vi "main(Test DQMH modules).bak.vi"() -> ()   [LabVIEW 2018, in "Application.lvlib"] (continued)
      frame "Test DRV 55" {
        w5444 = 55  # DUT index(0-59)
        n2417 = disable-structure shown="LOGGING==TRUE" {
          disable-tunnel: w5445 -> [w5480 _]
          frame condition #0 (active) {
            n2418 = Empty String/Path?(string/path=w5480) -> (empty?=w5483:bool)
            n2419 = Select(t="Quece timeout", s=w5483, f=w5480) -> (s? t:f=w5479:string)
            n2420 = call "string log (SubVI).vi"("Enum"=enum16{"Init", "Log", "Read"}."Log", "state Name"=w5479) -> ()  [unwired: 8 in, 2 out]
          }
          frame condition #1 {
          }
        }
        n2421 = call "progress string(SubVI).vi"("String 3"=w5445, "String in"=w5446) -> ("String out"=w5447:string)  [unwired: 9 in]
        n2422 = call "FGV Driver Data.vi"("DUT index(1-60)"=w5444) -> ("DUT SC"=w5443:bool)  [unwired: 7 in, 3 out]
        n2423 = case shown="False" w5443 {
          tunnel: [w5472 _] -> w5452
          tunnel: w5449 -> [w5471 _]
          frame False {
            w5459 = T11 {"command"="", "command data"=variant} ("element")
            w5458 = "MEAS.mux6_1"
            n2424 = To Variant(anything=T4."mux6-1_channel0" ("mux6_1(3wires)_encode")) -> (Variant=w5457:variant)
            n2425 = To Variant(anything=T4."mux6_1_channel1_3" ("mux6_1(3wires)_encode")) -> (Variant=w5469:variant)
            n2426 = To Variant(anything=T4."mux6-1_channel1_2" ("mux6_1(3wires)_encode")) -> (Variant=w5467:variant)
            n2427 = Bundle By Name(cluster=w5459, "command"=w5458, "command data"=w5467) -> (w5466:T11)
            n2428 = Bundle By Name(cluster=w5459, "command"=w5458, "command data"=w5469) -> (w5465:T11)
            n2429 = Bundle By Name(cluster=w5459, "command"=w5458, "command data"=w5457) -> ()  [unwired: 1 out]
            n2430 = Bundle By Name(cluster=w5459, "command"="MEAS.DMM dual read") -> (w5463:T11)
            n2431 = Build Array(w5466, w5465, w5463) -> (w5461:T11[])
            n2432 = Reverse 1D Array(array=w5461) -> (reversed array=w5462:T11[])
            n2433 = for {
              tunnel: [w5478] -> w5472 mode=indexing
              tunnel: w5471 -> [w5477]
              tunnel: w5462 -> [w5476] mode=indexing
              n2434 = Unbundle By Name(w5476) -> ("command"=w5475:string, "command data"=w5474:variant)
              n2435 = call "App enquece.vi"("Priority Enquece"=TRUE, "command data"=w5474, "command"=w5475, "queue in"=w5477) -> ("error out"=w5478:errorcluster)  [unwired: 6 in, 1 out]
            }
          }
          frame True {
          }
        }
        n2436 = Merge Errors(w5450, w5452) -> (w5451:errorcluster)
      }
      frame "Test DRV 56" {
        w5485 = 56  # DUT index(0-59)
        n2437 = disable-structure shown="LOGGING==TRUE" {
          disable-tunnel: w5486 -> [w5521 _]
          frame condition #0 (active) {
            n2438 = Empty String/Path?(string/path=w5521) -> (empty?=w5524:bool)
            n2439 = Select(t="Quece timeout", s=w5524, f=w5521) -> (s? t:f=w5520:string)
            n2440 = call "string log (SubVI).vi"("Enum"=enum16{"Init", "Log", "Read"}."Log", "state Name"=w5520) -> ()  [unwired: 8 in, 2 out]
          }
          frame condition #1 {
          }
        }
        n2441 = call "progress string(SubVI).vi"("String 3"=w5486, "String in"=w5487) -> ("String out"=w5488:string)  [unwired: 9 in]
        n2442 = call "FGV Driver Data.vi"("DUT index(1-60)"=w5485) -> ("DUT SC"=w5484:bool)  [unwired: 7 in, 3 out]
        n2443 = case shown="False" w5484 {
          tunnel: [w5513 _] -> w5493
          tunnel: w5490 -> [w5512 _]
          frame False {
            w5500 = T11 {"command"="", "command data"=variant} ("element")
            w5499 = "MEAS.mux6_1"
            n2444 = To Variant(anything=T4."mux6-1_channel0" ("mux6_1(3wires)_encode")) -> (Variant=w5498:variant)
            n2445 = To Variant(anything=T4."mux6_1_channel2_3" ("mux6_1(3wires)_encode")) -> (Variant=w5510:variant)
            n2446 = To Variant(anything=T4."mux6_1_channel2_2" ("mux6_1(3wires)_encode")) -> (Variant=w5508:variant)
            n2447 = Bundle By Name(cluster=w5500, "command"=w5499, "command data"=w5508) -> (w5507:T11)
            n2448 = Bundle By Name(cluster=w5500, "command"=w5499, "command data"=w5510) -> (w5506:T11)
            n2449 = Bundle By Name(cluster=w5500, "command"=w5499, "command data"=w5498) -> ()  [unwired: 1 out]
            n2450 = Bundle By Name(cluster=w5500, "command"="MEAS.DMM dual read") -> (w5504:T11)
            n2451 = Build Array(w5507, w5506, w5504) -> (w5502:T11[])
            n2452 = Reverse 1D Array(array=w5502) -> (reversed array=w5503:T11[])
            n2453 = for {
              tunnel: [w5519] -> w5513 mode=indexing
              tunnel: w5512 -> [w5518]
              tunnel: w5503 -> [w5517] mode=indexing
              n2454 = Unbundle By Name(w5517) -> ("command"=w5516:string, "command data"=w5515:variant)
              n2455 = call "App enquece.vi"("Priority Enquece"=TRUE, "command data"=w5515, "command"=w5516, "queue in"=w5518) -> ("error out"=w5519:errorcluster)  [unwired: 6 in, 1 out]
            }
          }
          frame True {
          }
        }
        n2456 = Merge Errors(w5491, w5493) -> (w5492:errorcluster)
      }
      frame "Test DRV 57" {
        w5526 = 57  # DUT index(0-59)
        n2457 = disable-structure shown="LOGGING==TRUE" {
          disable-tunnel: w5527 -> [w5562 _]
          frame condition #0 (active) {
            n2458 = Empty String/Path?(string/path=w5562) -> (empty?=w5565:bool)
            n2459 = Select(t="Quece timeout", s=w5565, f=w5562) -> (s? t:f=w5561:string)
            n2460 = call "string log (SubVI).vi"("Enum"=enum16{"Init", "Log", "Read"}."Log", "state Name"=w5561) -> ()  [unwired: 8 in, 2 out]
          }
          frame condition #1 {
          }
        }
        n2461 = call "progress string(SubVI).vi"("String 3"=w5527, "String in"=w5528) -> ("String out"=w5529:string)  [unwired: 9 in]
        n2462 = call "FGV Driver Data.vi"("DUT index(1-60)"=w5526) -> ("DUT SC"=w5525:bool)  [unwired: 7 in, 3 out]
        n2463 = case shown="False" w5525 {
          tunnel: [w5554 _] -> w5534
          tunnel: w5531 -> [w5553 _]
          frame False {
            w5541 = T11 {"command"="", "command data"=variant} ("element")
            w5540 = "MEAS.mux6_1"
            n2464 = To Variant(anything=T4."mux6-1_channel0" ("mux6_1(3wires)_encode")) -> (Variant=w5539:variant)
            n2465 = To Variant(anything=T4."mux6_1_channel3_3" ("mux6_1(3wires)_encode")) -> (Variant=w5551:variant)
            n2466 = To Variant(anything=T4."mux6_1_channel3_2" ("mux6_1(3wires)_encode")) -> (Variant=w5549:variant)
            n2467 = Bundle By Name(cluster=w5541, "command"=w5540, "command data"=w5549) -> (w5548:T11)
            n2468 = Bundle By Name(cluster=w5541, "command"=w5540, "command data"=w5551) -> (w5547:T11)
            n2469 = Bundle By Name(cluster=w5541, "command"=w5540, "command data"=w5539) -> ()  [unwired: 1 out]
            n2470 = Bundle By Name(cluster=w5541, "command"="MEAS.DMM dual read") -> (w5545:T11)
            n2471 = Build Array(w5548, w5547, w5545) -> (w5543:T11[])
            n2472 = Reverse 1D Array(array=w5543) -> (reversed array=w5544:T11[])
            n2473 = for {
              tunnel: [w5560] -> w5554 mode=indexing
              tunnel: w5553 -> [w5559]
              tunnel: w5544 -> [w5558] mode=indexing
              n2474 = Unbundle By Name(w5558) -> ("command"=w5557:string, "command data"=w5556:variant)
              n2475 = call "App enquece.vi"("Priority Enquece"=TRUE, "command data"=w5556, "command"=w5557, "queue in"=w5559) -> ("error out"=w5560:errorcluster)  [unwired: 6 in, 1 out]
            }
          }
          frame True {
          }
        }
        n2476 = Merge Errors(w5532, w5534) -> (w5533:errorcluster)
      }
      frame "Test DRV 58" {
        w5567 = 58  # DUT index(0-59)
        n2477 = disable-structure shown="LOGGING==TRUE" {
          disable-tunnel: w5568 -> [w5603 _]
          frame condition #0 (active) {
            n2478 = Empty String/Path?(string/path=w5603) -> (empty?=w5606:bool)
            n2479 = Select(t="Quece timeout", s=w5606, f=w5603) -> (s? t:f=w5602:string)
            n2480 = call "string log (SubVI).vi"("Enum"=enum16{"Init", "Log", "Read"}."Log", "state Name"=w5602) -> ()  [unwired: 8 in, 2 out]
          }
          frame condition #1 {
          }
        }
        n2481 = call "progress string(SubVI).vi"("String 3"=w5568, "String in"=w5569) -> ("String out"=w5570:string)  [unwired: 9 in]
        n2482 = call "FGV Driver Data.vi"("DUT index(1-60)"=w5567) -> ("DUT SC"=w5566:bool)  [unwired: 7 in, 3 out]
        n2483 = case shown="False" w5566 {
          tunnel: [w5595 _] -> w5575
          tunnel: w5572 -> [w5594 _]
          frame False {
            w5582 = T11 {"command"="", "command data"=variant} ("element")
            w5581 = "MEAS.mux6_1"
            n2484 = To Variant(anything=T4."mux6-1_channel0" ("mux6_1(3wires)_encode")) -> (Variant=w5580:variant)
            n2485 = To Variant(anything=T4."mux6_1_channel4_3" ("mux6_1(3wires)_encode")) -> (Variant=w5592:variant)
            n2486 = To Variant(anything=T4."mux6_1_channel4_2" ("mux6_1(3wires)_encode")) -> (Variant=w5590:variant)
            n2487 = Bundle By Name(cluster=w5582, "command"=w5581, "command data"=w5590) -> (w5589:T11)
            n2488 = Bundle By Name(cluster=w5582, "command"=w5581, "command data"=w5592) -> (w5588:T11)
            n2489 = Bundle By Name(cluster=w5582, "command"=w5581, "command data"=w5580) -> ()  [unwired: 1 out]
            n2490 = Bundle By Name(cluster=w5582, "command"="MEAS.DMM dual read") -> (w5586:T11)
            n2491 = Build Array(w5589, w5588, w5586) -> (w5584:T11[])
            n2492 = Reverse 1D Array(array=w5584) -> (reversed array=w5585:T11[])
            n2493 = for {
              tunnel: [w5601] -> w5595 mode=indexing
              tunnel: w5594 -> [w5600]
              tunnel: w5585 -> [w5599] mode=indexing
              n2494 = Unbundle By Name(w5599) -> ("command"=w5598:string, "command data"=w5597:variant)
              n2495 = call "App enquece.vi"("Priority Enquece"=TRUE, "command data"=w5597, "command"=w5598, "queue in"=w5600) -> ("error out"=w5601:errorcluster)  [unwired: 6 in, 1 out]
            }
          }
          frame True {
          }
        }
        n2496 = Merge Errors(w5573, w5575) -> (w5574:errorcluster)
      }
      frame "Test DRV 59" {
        w5608 = 59  # DUT index(0-59)
        n2497 = disable-structure shown="LOGGING==TRUE" {
          disable-tunnel: w5609 -> [w5644 _]
          frame condition #0 (active) {
            n2498 = Empty String/Path?(string/path=w5644) -> (empty?=w5647:bool)
            n2499 = Select(t="Quece timeout", s=w5647, f=w5644) -> (s? t:f=w5643:string)
            n2500 = call "string log (SubVI).vi"("Enum"=enum16{"Init", "Log", "Read"}."Log", "state Name"=w5643) -> ()  [unwired: 8 in, 2 out]
          }
          frame condition #1 {
          }
        }
        n2501 = call "progress string(SubVI).vi"("String 3"=w5609, "String in"=w5610) -> ("String out"=w5611:string)  [unwired: 9 in]
        n2502 = call "FGV Driver Data.vi"("DUT index(1-60)"=w5608) -> ("DUT SC"=w5607:bool)  [unwired: 7 in, 3 out]
        n2503 = case shown="False" w5607 {
          tunnel: [w5636 _] -> w5616
          tunnel: w5613 -> [w5635 _]
          frame False {
            w5623 = T11 {"command"="", "command data"=variant} ("element")
            w5622 = "MEAS.mux6_1"
            n2504 = To Variant(anything=T4."mux6-1_channel0" ("mux6_1(3wires)_encode")) -> (Variant=w5621:variant)
            n2505 = To Variant(anything=T4."mux6_1_channel5_3" ("mux6_1(3wires)_encode")) -> (Variant=w5633:variant)
            n2506 = To Variant(anything=T4."mux6_1_channel5_2" ("mux6_1(3wires)_encode")) -> (Variant=w5631:variant)
            n2507 = Bundle By Name(cluster=w5623, "command"=w5622, "command data"=w5631) -> (w5630:T11)
            n2508 = Bundle By Name(cluster=w5623, "command"=w5622, "command data"=w5633) -> (w5629:T11)
            n2509 = Bundle By Name(cluster=w5623, "command"=w5622, "command data"=w5621) -> ()  [unwired: 1 out]
            n2510 = Bundle By Name(cluster=w5623, "command"="MEAS.DMM dual read") -> (w5627:T11)
            n2511 = Build Array(w5630, w5629, w5627) -> (w5625:T11[])
            n2512 = Reverse 1D Array(array=w5625) -> (reversed array=w5626:T11[])
            n2513 = for {
              tunnel: [w5642] -> w5636 mode=indexing
              tunnel: w5635 -> [w5641]
              tunnel: w5626 -> [w5640] mode=indexing
              n2514 = Unbundle By Name(w5640) -> ("command"=w5639:string, "command data"=w5638:variant)
              n2515 = call "App enquece.vi"("Priority Enquece"=TRUE, "command data"=w5638, "command"=w5639, "queue in"=w5641) -> ("error out"=w5642:errorcluster)  [unwired: 6 in, 1 out]
            }
          }
          frame True {
          }
        }
        n2516 = Merge Errors(w5614, w5616) -> (w5615:errorcluster)
      }
      frame "Test DRV 60" {
        w5649 = 60  # DUT index(0-59)
        n2517 = disable-structure shown="LOGGING==TRUE" {
          disable-tunnel: w5650 -> [w5685 _]
          frame condition #0 (active) {
            n2518 = Empty String/Path?(string/path=w5685) -> (empty?=w5688:bool)
            n2519 = Select(t="Quece timeout", s=w5688, f=w5685) -> (s? t:f=w5684:string)
            n2520 = call "string log (SubVI).vi"("Enum"=enum16{"Init", "Log", "Read"}."Log", "state Name"=w5684) -> ()  [unwired: 8 in, 2 out]
          }
          frame condition #1 {
          }
        }
        n2521 = call "progress string(SubVI).vi"("String 3"=w5650, "String in"=w5651) -> ("String out"=w5652:string)  [unwired: 9 in]
        n2522 = call "FGV Driver Data.vi"("DUT index(1-60)"=w5649) -> ("DUT SC"=w5648:bool)  [unwired: 7 in, 3 out]
        n2523 = case shown="True" w5648 {
          tunnel: [w5677 _] -> w5657
          tunnel: w5654 -> [w5676 _]
          frame False {
            w5664 = T11 {"command"="", "command data"=variant} ("element")
            w5663 = "MEAS.mux6_1"
            n2524 = To Variant(anything=T4."mux6-1_channel0" ("mux6_1(3wires)_encode")) -> (Variant=w5662:variant)
            n2525 = To Variant(anything=T4."mux6_1_channel6_3" ("mux6_1(3wires)_encode")) -> (Variant=w5674:variant)
            n2526 = To Variant(anything=T4."mux6_1_channel6_2" ("mux6_1(3wires)_encode")) -> (Variant=w5672:variant)
            n2527 = Bundle By Name(cluster=w5664, "command"=w5663, "command data"=w5672) -> (w5671:T11)
            n2528 = Bundle By Name(cluster=w5664, "command"=w5663, "command data"=w5674) -> (w5670:T11)
            n2529 = Bundle By Name(cluster=w5664, "command"=w5663, "command data"=w5662) -> ()  [unwired: 1 out]
            n2530 = Bundle By Name(cluster=w5664, "command"="MEAS.DMM dual read") -> (w5668:T11)
            n2531 = Build Array(w5671, w5670, w5668) -> (w5666:T11[])
            n2532 = Reverse 1D Array(array=w5666) -> (reversed array=w5667:T11[])
            n2533 = for {
              tunnel: [w5683] -> w5677 mode=indexing
              tunnel: w5676 -> [w5682]
              tunnel: w5667 -> [w5681] mode=indexing
              n2534 = Unbundle By Name(w5681) -> ("command"=w5680:string, "command data"=w5679:variant)
              n2535 = call "App enquece.vi"("Priority Enquece"=TRUE, "command data"=w5679, "command"=w5680, "queue in"=w5682) -> ("error out"=w5683:errorcluster)  [unwired: 6 in, 1 out]
            }
          }
          frame True {
          }
        }
        n2536 = Merge Errors(w5655, w5657) -> (w5656:errorcluster)
      }
      frame "separated" {
      }
      frame "Test DRV 1A" {
        w5703 = T11 {"command"="", "command data"=variant} ("element")
        w5698 = 1 ("DUT index(0-59)")
        w5729 = T11 {"command"="", "command data"=variant} ("element")
        n2537 = disable-structure shown="LOGGING==TRUE" {
          disable-tunnel: w5707 -> [w5745 _]
          frame condition #0 (active) {
            n2538 = Empty String/Path?(string/path=w5745) -> (empty?=w5748:bool)
            n2539 = Select(t="Quece timeout", s=w5748, f=w5745) -> (s? t:f=w5744:string)
            n2540 = call "string log (SubVI).vi"("Enum"=enum16{"Init", "Log", "Read"}."Log", "state Name"=w5744) -> ()  [unwired: 8 in, 2 out]
          }
          frame condition #1 {
          }
        }
        n2541 = Flush Queue(queue=w5708) -> (queue out=w5709:refnum<queue>)  [unwired: 1 in, 2 out]
        n2542 = Decrement(x=w5698) -> (x-1=w5701:i32)
        n2543 = Index Array(array=w5697, index=w5701) -> (element=w5699:refnum<vi>)
        n2544 = property class="ColBox"(reference=w5699, "Value"=u32 10000536 ("DRV 1")) -> ()  [unwired: 1 in, 2 out]
        n2545 = To Variant(anything=bool[] [TRUE, FALSE, FALSE, FALSE, FALSE, FALSE]) -> (Variant=w5726:variant)
        n2546 = To Variant(anything=T6."demux1_10_channel1" ("demux1_10(x6)_encode")) -> (Variant=w5730:variant)
        n2547 = To Variant(anything=T4."mux6_1_channel1_3" ("mux6_1(3wires)_encode")) -> (Variant=w5734:variant)
        n2548 = To Variant(anything=T5."mux10_1_channel1" ("mux10_1(x6)_encode")) -> (Variant=w5736:variant)
        n2549 = Bundle By Name(cluster=w5729, "command"="MEAS.mux10-1", "command data"=w5736) -> (w5724:T11)
        n2550 = Bundle By Name(cluster=w5729, "command"="MEAS.mux6_1", "command data"=w5734) -> (w5723:T11)
        n2551 = Bundle By Name(cluster=w5729, "command"="MEAS.demux1-10", "command data"=w5730) -> (w5722:T11)
        n2552 = Bundle By Name(cluster=w5729, "command"="MEAS.eMIC", "command data"=w5726) -> (w5721:T11)
        n2553 = Bundle By Name(cluster=w5729, "command"="MEAS.AllRelaysOFF") -> (w5725:T11)
        n2554 = Build Array(w5725, w5724, w5723, w5722, w5721) -> (w5716:T11[])
        n2555 = Bundle By Name(cluster=w5703, "command"="MEAS.requestAC", "command data"=w5698) -> (w5717:T11)
        n2556 = Bundle By Name(cluster=w5703, "command"="Apps.WaitForEvent", "command data"=w5698) -> (w5702:T11)
        n2557 = Bundle By Name(cluster=w5703, "command"="MEAS.DMM dual read") -> (w5718:T11)
        n2558 = Bundle By Name(cluster=w5703, "command"="Apps.UI Update 1") -> (w5704:T11)
        n2559 = Build Array(w5718, w5717, w5702, w5704) -> (w5715:T11[])
        n2560 = Build Array (concatenate)(w5716, w5715) -> (w5714:T11[])
        n2561 = for {
          tunnel: w5714 -> [w5752] mode=indexing
          tunnel: w5709 -> [w5753]
          tunnel: [w5749] -> w5712 mode=indexing
          n2562 = Unbundle By Name(w5752) -> ("command"=w5751:string, "command data"=w5750:variant)
          n2563 = call "App enquece.vi"("command data"=w5750, "command"=w5751, "queue in"=w5753) -> ("error out"=w5749:errorcluster)  [unwired: 7 in, 1 out]
        }
        n2564 = Merge Errors(w5713, w5712) -> (w5711:errorcluster)
      }
      frame "Test DRV 2A" {
        w5760 = T11 {"command"="", "command data"=variant} ("element")
        w5755 = 2 ("DUT index(0-59)")
        w5786 = T11 {"command"="", "command data"=variant} ("element")
        n2565 = disable-structure shown="LOGGING==TRUE" {
          disable-tunnel: w5764 -> [w5802 _]
          frame condition #0 (active) {
            n2566 = Empty String/Path?(string/path=w5802) -> (empty?=w5805:bool)
            n2567 = Select(t="Quece timeout", s=w5805, f=w5802) -> (s? t:f=w5801:string)
            n2568 = call "string log (SubVI).vi"("Enum"=enum16{"Init", "Log", "Read"}."Log", "state Name"=w5801) -> ()  [unwired: 8 in, 2 out]
          }
          frame condition #1 {
          }
        }
        n2569 = Flush Queue(queue=w5765) -> (queue out=w5766:refnum<queue>)  [unwired: 1 in, 2 out]
        n2570 = Decrement(x=w5755) -> (x-1=w5758:i32)
        n2571 = Index Array(array=w5754, index=w5758) -> (element=w5756:refnum<vi>)
        n2572 = property class="ColBox"(reference=w5756, "Value"=u32 10000536 ("DRV 1")) -> ()  [unwired: 1 in, 2 out]
        n2573 = To Variant(anything=bool[] [FALSE, TRUE, FALSE, FALSE, FALSE, FALSE]) -> (Variant=w5783:variant)
        n2574 = To Variant(anything=T6."demux1_10_channel1" ("demux1_10(x6)_encode")) -> (Variant=w5787:variant)
        n2575 = To Variant(anything=T4."mux6_1_channel2_3" ("mux6_1(3wires)_encode")) -> (Variant=w5791:variant)
        n2576 = To Variant(anything=T5."mux10_1_channel1" ("mux10_1(x6)_encode")) -> (Variant=w5793:variant)
        n2577 = Bundle By Name(cluster=w5786, "command"="MEAS.mux10-1", "command data"=w5793) -> (w5781:T11)
        n2578 = Bundle By Name(cluster=w5786, "command"="MEAS.mux6_1", "command data"=w5791) -> (w5780:T11)
        n2579 = Bundle By Name(cluster=w5786, "command"="MEAS.demux1-10", "command data"=w5787) -> (w5779:T11)
        n2580 = Bundle By Name(cluster=w5786, "command"="MEAS.eMIC", "command data"=w5783) -> (w5778:T11)
        n2581 = Bundle By Name(cluster=w5786, "command"="MEAS.AllRelaysOFF") -> (w5782:T11)
        n2582 = Build Array(w5782, w5781, w5780, w5779, w5778) -> (w5773:T11[])
        n2583 = Bundle By Name(cluster=w5760, "command"="MEAS.requestAC", "command data"=w5755) -> (w5774:T11)
        n2584 = Bundle By Name(cluster=w5760, "command"="Apps.WaitForEvent", "command data"=w5755) -> (w5759:T11)
        n2585 = Bundle By Name(cluster=w5760, "command"="MEAS.DMM dual read") -> (w5775:T11)
        n2586 = Bundle By Name(cluster=w5760, "command"="Apps.UI Update 1") -> (w5761:T11)
        n2587 = Build Array(w5775, w5774, w5759, w5761) -> (w5772:T11[])
        n2588 = Build Array (concatenate)(w5773, w5772) -> (w5771:T11[])
        n2589 = for {
          tunnel: w5771 -> [w5809] mode=indexing
          tunnel: w5766 -> [w5810]
          tunnel: [w5806] -> w5769 mode=indexing
          n2590 = Unbundle By Name(w5809) -> ("command"=w5808:string, "command data"=w5807:variant)
          n2591 = call "App enquece.vi"("command data"=w5807, "command"=w5808, "queue in"=w5810) -> ("error out"=w5806:errorcluster)  [unwired: 7 in, 1 out]
        }
        n2592 = Merge Errors(w5770, w5769) -> (w5768:errorcluster)
      }
      frame "Test DRV 3A" {
        w5817 = T11 {"command"="", "command data"=variant} ("element")
        w5812 = 3 ("DUT index(0-59)")
        w5843 = T11 {"command"="", "command data"=variant} ("element")
        n2593 = disable-structure shown="LOGGING==TRUE" {
          disable-tunnel: w5821 -> [w5859 _]
          frame condition #0 (active) {
            n2594 = Empty String/Path?(string/path=w5859) -> (empty?=w5862:bool)
            n2595 = Select(t="Quece timeout", s=w5862, f=w5859) -> (s? t:f=w5858:string)
            n2596 = call "string log (SubVI).vi"("Enum"=enum16{"Init", "Log", "Read"}."Log", "state Name"=w5858) -> ()  [unwired: 8 in, 2 out]
          }
          frame condition #1 {
          }
        }
        n2597 = Flush Queue(queue=w5822) -> (queue out=w5823:refnum<queue>)  [unwired: 1 in, 2 out]
        n2598 = Decrement(x=w5812) -> (x-1=w5815:i32)
        n2599 = Index Array(array=w5811, index=w5815) -> (element=w5813:refnum<vi>)
        n2600 = property class="ColBox"(reference=w5813, "Value"=u32 10000536 ("DRV 1")) -> ()  [unwired: 1 in, 2 out]
        n2601 = To Variant(anything=bool[] [FALSE, FALSE, TRUE, FALSE, FALSE, FALSE]) -> (Variant=w5840:variant)
        n2602 = To Variant(anything=T6."demux1_10_channel1" ("demux1_10(x6)_encode")) -> (Variant=w5844:variant)
        n2603 = To Variant(anything=T4."mux6_1_channel3_3" ("mux6_1(3wires)_encode")) -> (Variant=w5848:variant)
        n2604 = To Variant(anything=T5."mux10_1_channel1" ("mux10_1(x6)_encode")) -> (Variant=w5850:variant)
        n2605 = Bundle By Name(cluster=w5843, "command"="MEAS.mux10-1", "command data"=w5850) -> (w5838:T11)
        n2606 = Bundle By Name(cluster=w5843, "command"="MEAS.mux6_1", "command data"=w5848) -> (w5837:T11)
        n2607 = Bundle By Name(cluster=w5843, "command"="MEAS.demux1-10", "command data"=w5844) -> (w5836:T11)
        n2608 = Bundle By Name(cluster=w5843, "command"="MEAS.eMIC", "command data"=w5840) -> (w5835:T11)
        n2609 = Bundle By Name(cluster=w5843, "command"="MEAS.AllRelaysOFF") -> (w5839:T11)
        n2610 = Build Array(w5839, w5838, w5837, w5836, w5835) -> (w5830:T11[])
        n2611 = Bundle By Name(cluster=w5817, "command"="MEAS.requestAC", "command data"=w5812) -> (w5831:T11)
        n2612 = Bundle By Name(cluster=w5817, "command"="Apps.WaitForEvent", "command data"=w5812) -> (w5816:T11)
        n2613 = Bundle By Name(cluster=w5817, "command"="MEAS.DMM dual read") -> (w5832:T11)
        n2614 = Bundle By Name(cluster=w5817, "command"="Apps.UI Update 1") -> (w5818:T11)
        n2615 = Build Array(w5832, w5831, w5816, w5818) -> (w5829:T11[])
        n2616 = Build Array (concatenate)(w5830, w5829) -> (w5828:T11[])
        n2617 = for {
          tunnel: w5828 -> [w5866] mode=indexing
          tunnel: w5823 -> [w5867]
          tunnel: [w5863] -> w5826 mode=indexing
          n2618 = Unbundle By Name(w5866) -> ("command"=w5865:string, "command data"=w5864:variant)
          n2619 = call "App enquece.vi"("command data"=w5864, "command"=w5865, "queue in"=w5867) -> ("error out"=w5863:errorcluster)  [unwired: 7 in, 1 out]
        }
        n2620 = Merge Errors(w5827, w5826) -> (w5825:errorcluster)
      }
      frame "Test DRV 4A" {
        w5874 = T11 {"command"="", "command data"=variant} ("element")
        w5868 = 4 ("DUT index(0-59)")
        w5900 = T11 {"command"="", "command data"=variant} ("element")
        n2621 = disable-structure shown="LOGGING==TRUE" {
          disable-tunnel: w5878 -> [w5916 _]
          frame condition #0 (active) {
            n2622 = Empty String/Path?(string/path=w5916) -> (empty?=w5919:bool)
            n2623 = Select(t="Quece timeout", s=w5919, f=w5916) -> (s? t:f=w5915:string)
            n2624 = call "string log (SubVI).vi"("Enum"=enum16{"Init", "Log", "Read"}."Log", "state Name"=w5915) -> ()  [unwired: 8 in, 2 out]
          }
          frame condition #1 {
          }
        }
        n2625 = Flush Queue(queue=w5879) -> (queue out=w5880:refnum<queue>)  [unwired: 1 in, 2 out]
        n2626 = Decrement(x=w5868) -> (x-1=w5872:i32)
        n2627 = Index Array(array=w5869, index=w5872) -> (element=w5870:refnum<vi>)
        n2628 = property class="ColBox"(reference=w5870, "Value"=u32 10000536 ("DRV 1")) -> ()  [unwired: 1 in, 2 out]
        n2629 = To Variant(anything=bool[] [FALSE, FALSE, FALSE, TRUE, FALSE, FALSE]) -> (Variant=w5897:variant)
        n2630 = To Variant(anything=T6."demux1_10_channel1" ("demux1_10(x6)_encode")) -> (Variant=w5901:variant)
        n2631 = To Variant(anything=T4."mux6_1_channel4_3" ("mux6_1(3wires)_encode")) -> (Variant=w5905:variant)
        n2632 = To Variant(anything=T5."mux10_1_channel1" ("mux10_1(x6)_encode")) -> (Variant=w5907:variant)
        n2633 = Bundle By Name(cluster=w5900, "command"="MEAS.mux10-1", "command data"=w5907) -> (w5895:T11)
        n2634 = Bundle By Name(cluster=w5900, "command"="MEAS.mux6_1", "command data"=w5905) -> (w5894:T11)
        n2635 = Bundle By Name(cluster=w5900, "command"="MEAS.demux1-10", "command data"=w5901) -> (w5893:T11)
        n2636 = Bundle By Name(cluster=w5900, "command"="MEAS.eMIC", "command data"=w5897) -> (w5892:T11)
        n2637 = Bundle By Name(cluster=w5900, "command"="MEAS.AllRelaysOFF") -> (w5896:T11)
        n2638 = Build Array(w5896, w5895, w5894, w5893, w5892) -> (w5887:T11[])
        n2639 = Bundle By Name(cluster=w5874, "command"="MEAS.requestAC", "command data"=w5868) -> (w5888:T11)
        n2640 = Bundle By Name(cluster=w5874, "command"="Apps.WaitForEvent", "command data"=w5868) -> (w5873:T11)
        n2641 = Bundle By Name(cluster=w5874, "command"="MEAS.DMM dual read") -> (w5889:T11)
        n2642 = Bundle By Name(cluster=w5874, "command"="Apps.UI Update 1") -> (w5875:T11)
        n2643 = Build Array(w5889, w5888, w5873, w5875) -> (w5886:T11[])
        n2644 = Build Array (concatenate)(w5887, w5886) -> (w5885:T11[])
        n2645 = for {
          tunnel: w5885 -> [w5923] mode=indexing
          tunnel: w5880 -> [w5924]
          tunnel: [w5920] -> w5883 mode=indexing
          n2646 = Unbundle By Name(w5923) -> ("command"=w5922:string, "command data"=w5921:variant)
          n2647 = call "App enquece.vi"("command data"=w5921, "command"=w5922, "queue in"=w5924) -> ("error out"=w5920:errorcluster)  [unwired: 7 in, 1 out]
        }
        n2648 = Merge Errors(w5884, w5883) -> (w5882:errorcluster)
      }
      frame "Test DRV 5A" {
        w5931 = T11 {"command"="", "command data"=variant} ("element")
        w5926 = 5 ("DUT index(0-59)")
        w5957 = T11 {"command"="", "command data"=variant} ("element")
        n2649 = disable-structure shown="LOGGING==TRUE" {
          disable-tunnel: w5935 -> [w5973 _]
          frame condition #0 (active) {
            n2650 = Empty String/Path?(string/path=w5973) -> (empty?=w5976:bool)
            n2651 = Select(t="Quece timeout", s=w5976, f=w5973) -> (s? t:f=w5972:string)
            n2652 = call "string log (SubVI).vi"("Enum"=enum16{"Init", "Log", "Read"}."Log", "state Name"=w5972) -> ()  [unwired: 8 in, 2 out]
          }
          frame condition #1 {
          }
        }
        n2653 = Flush Queue(queue=w5936) -> (queue out=w5937:refnum<queue>)  [unwired: 1 in, 2 out]
        n2654 = Decrement(x=w5926) -> (x-1=w5929:i32)
        n2655 = Index Array(array=w5925, index=w5929) -> (element=w5927:refnum<vi>)
        n2656 = property class="ColBox"(reference=w5927, "Value"=u32 10000536 ("DRV 1")) -> ()  [unwired: 1 in, 2 out]
        n2657 = To Variant(anything=bool[] [FALSE, FALSE, FALSE, FALSE, TRUE, FALSE]) -> (Variant=w5954:variant)
        n2658 = To Variant(anything=T6."demux1_10_channel1" ("demux1_10(x6)_encode")) -> (Variant=w5958:variant)
        n2659 = To Variant(anything=T4."mux6_1_channel5_3" ("mux6_1(3wires)_encode")) -> (Variant=w5962:variant)
        n2660 = To Variant(anything=T5."mux10_1_channel1" ("mux10_1(x6)_encode")) -> (Variant=w5964:variant)
        n2661 = Bundle By Name(cluster=w5957, "command"="MEAS.mux10-1", "command data"=w5964) -> (w5952:T11)
        n2662 = Bundle By Name(cluster=w5957, "command"="MEAS.mux6_1", "command data"=w5962) -> (w5951:T11)
        n2663 = Bundle By Name(cluster=w5957, "command"="MEAS.demux1-10", "command data"=w5958) -> (w5950:T11)
        n2664 = Bundle By Name(cluster=w5957, "command"="MEAS.eMIC", "command data"=w5954) -> (w5949:T11)
        n2665 = Bundle By Name(cluster=w5957, "command"="MEAS.AllRelaysOFF") -> (w5953:T11)
        n2666 = Build Array(w5953, w5952, w5951, w5950, w5949) -> (w5944:T11[])
        n2667 = Bundle By Name(cluster=w5931, "command"="MEAS.requestAC", "command data"=w5926) -> (w5945:T11)
        n2668 = Bundle By Name(cluster=w5931, "command"="Apps.WaitForEvent", "command data"=w5926) -> (w5930:T11)
        n2669 = Bundle By Name(cluster=w5931, "command"="MEAS.DMM dual read") -> (w5946:T11)
        n2670 = Bundle By Name(cluster=w5931, "command"="Apps.UI Update 1") -> (w5932:T11)
        n2671 = Build Array(w5946, w5945, w5930, w5932) -> (w5943:T11[])
        n2672 = Build Array (concatenate)(w5944, w5943) -> (w5942:T11[])
        n2673 = for {
          tunnel: w5942 -> [w5980] mode=indexing
          tunnel: w5937 -> [w5981]
          tunnel: [w5977] -> w5940 mode=indexing
          n2674 = Unbundle By Name(w5980) -> ("command"=w5979:string, "command data"=w5978:variant)
          n2675 = call "App enquece.vi"("command data"=w5978, "command"=w5979, "queue in"=w5981) -> ("error out"=w5977:errorcluster)  [unwired: 7 in, 1 out]
        }
        n2676 = Merge Errors(w5941, w5940) -> (w5939:errorcluster)
      }
      frame "Test DRV 6A" {
        w5988 = T11 {"command"="", "command data"=variant} ("element")
        w5982 = 6 ("DUT index(0-59)")
        w6014 = T11 {"command"="", "command data"=variant} ("element")
        n2677 = disable-structure shown="LOGGING==TRUE" {
          disable-tunnel: w5992 -> [w6030 _]
          frame condition #0 (active) {
            n2678 = Empty String/Path?(string/path=w6030) -> (empty?=w6033:bool)
            n2679 = Select(t="Quece timeout", s=w6033, f=w6030) -> (s? t:f=w6029:string)
            n2680 = call "string log (SubVI).vi"("Enum"=enum16{"Init", "Log", "Read"}."Log", "state Name"=w6029) -> ()  [unwired: 8 in, 2 out]
          }
          frame condition #1 {
          }
        }
        n2681 = Flush Queue(queue=w5993) -> (queue out=w5994:refnum<queue>)  [unwired: 1 in, 2 out]
        n2682 = Decrement(x=w5982) -> (x-1=w5986:i32)
        n2683 = Index Array(array=w5983, index=w5986) -> (element=w5984:refnum<vi>)
        n2684 = property class="ColBox"(reference=w5984, "Value"=u32 10000536 ("DRV 1")) -> ()  [unwired: 1 in, 2 out]
        n2685 = To Variant(anything=bool[] [FALSE, FALSE, FALSE, FALSE, FALSE, TRUE]) -> (Variant=w6011:variant)
        n2686 = To Variant(anything=T6."demux1_10_channel1" ("demux1_10(x6)_encode")) -> (Variant=w6015:variant)
        n2687 = To Variant(anything=T4."mux6_1_channel5_3" ("mux6_1(3wires)_encode")) -> (Variant=w6019:variant)
        n2688 = To Variant(anything=T5."mux10_1_channel1" ("mux10_1(x6)_encode")) -> (Variant=w6021:variant)
        n2689 = Bundle By Name(cluster=w6014, "command"="MEAS.mux10-1", "command data"=w6021) -> (w6009:T11)
        n2690 = Bundle By Name(cluster=w6014, "command"="MEAS.mux6_1", "command data"=w6019) -> (w6008:T11)
        n2691 = Bundle By Name(cluster=w6014, "command"="MEAS.demux1-10", "command data"=w6015) -> (w6007:T11)
        n2692 = Bundle By Name(cluster=w6014, "command"="MEAS.eMIC", "command data"=w6011) -> (w6006:T11)
        n2693 = Bundle By Name(cluster=w6014, "command"="MEAS.AllRelaysOFF") -> (w6010:T11)
        n2694 = Build Array(w6010, w6009, w6008, w6007, w6006) -> (w6001:T11[])
        n2695 = Bundle By Name(cluster=w5988, "command"="MEAS.requestAC", "command data"=w5982) -> (w6002:T11)
        n2696 = Bundle By Name(cluster=w5988, "command"="Apps.WaitForEvent", "command data"=w5982) -> (w5987:T11)
        n2697 = Bundle By Name(cluster=w5988, "command"="MEAS.DMM dual read") -> (w6003:T11)
        n2698 = Bundle By Name(cluster=w5988, "command"="Apps.UI Update 1") -> (w5989:T11)
        n2699 = Build Array(w6003, w6002, w5987, w5989) -> (w6000:T11[])
        n2700 = Build Array (concatenate)(w6001, w6000) -> (w5999:T11[])
        n2701 = for {
          tunnel: w5999 -> [w6037] mode=indexing
          tunnel: w5994 -> [w6038]
          tunnel: [w6034] -> w5997 mode=indexing
          n2702 = Unbundle By Name(w6037) -> ("command"=w6036:string, "command data"=w6035:variant)
          n2703 = call "App enquece.vi"("command data"=w6035, "command"=w6036, "queue in"=w6038) -> ("error out"=w6034:errorcluster)  [unwired: 7 in, 1 out]
        }
        n2704 = Merge Errors(w5998, w5997) -> (w5996:errorcluster)
      }
      frame "Test DRV 7A" {
        w6045 = T11 {"command"="", "command data"=variant} ("element")
        w6039 = 7 ("DUT index(0-59)")
        w6071 = T11 {"command"="", "command data"=variant} ("element")
        n2705 = disable-structure shown="LOGGING==TRUE" {
          disable-tunnel: w6049 -> [w6087 _]
          frame condition #0 (active) {
            n2706 = Empty String/Path?(string/path=w6087) -> (empty?=w6090:bool)
            n2707 = Select(t="Quece timeout", s=w6090, f=w6087) -> (s? t:f=w6086:string)
            n2708 = call "string log (SubVI).vi"("Enum"=enum16{"Init", "Log", "Read"}."Log", "state Name"=w6086) -> ()  [unwired: 8 in, 2 out]
          }
          frame condition #1 {
          }
        }
        n2709 = Flush Queue(queue=w6050) -> (queue out=w6051:refnum<queue>)  [unwired: 1 in, 2 out]
        n2710 = Decrement(x=w6039) -> (x-1=w6043:i32)
        n2711 = Index Array(array=w6040, index=w6043) -> (element=w6041:refnum<vi>)
        n2712 = property class="ColBox"(reference=w6041, "Value"=u32 10000536 ("DRV 1")) -> ()  [unwired: 1 in, 2 out]
        n2713 = To Variant(anything=bool[] [TRUE, FALSE, FALSE, FALSE, FALSE, FALSE]) -> (Variant=w6068:variant)
        n2714 = To Variant(anything=T6."demux1_10_channel2" ("demux1_10(x6)_encode")) -> (Variant=w6072:variant)
        n2715 = To Variant(anything=T4."mux6_1_channel1_3" ("mux6_1(3wires)_encode")) -> (Variant=w6076:variant)
        n2716 = To Variant(anything=T5."mux10_1_channel2" ("mux10_1(x6)_encode")) -> (Variant=w6078:variant)
        n2717 = Bundle By Name(cluster=w6071, "command"="MEAS.mux10-1", "command data"=w6078) -> (w6066:T11)
        n2718 = Bundle By Name(cluster=w6071, "command"="MEAS.mux6_1", "command data"=w6076) -> (w6065:T11)
        n2719 = Bundle By Name(cluster=w6071, "command"="MEAS.demux1-10", "command data"=w6072) -> (w6064:T11)
        n2720 = Bundle By Name(cluster=w6071, "command"="MEAS.eMIC", "command data"=w6068) -> (w6063:T11)
        n2721 = Bundle By Name(cluster=w6071, "command"="MEAS.AllRelaysOFF") -> (w6067:T11)
        n2722 = Build Array(w6067, w6066, w6065, w6064, w6063) -> (w6058:T11[])
        n2723 = Bundle By Name(cluster=w6045, "command"="MEAS.requestAC", "command data"=w6039) -> (w6059:T11)
        n2724 = Bundle By Name(cluster=w6045, "command"="Apps.WaitForEvent", "command data"=w6039) -> (w6044:T11)
        n2725 = Bundle By Name(cluster=w6045, "command"="MEAS.DMM dual read") -> (w6060:T11)
        n2726 = Bundle By Name(cluster=w6045, "command"="Apps.UI Update 1") -> (w6046:T11)
        n2727 = Build Array(w6060, w6059, w6044, w6046) -> (w6057:T11[])
        n2728 = Build Array (concatenate)(w6058, w6057) -> (w6056:T11[])
        n2729 = for {
          tunnel: w6056 -> [w6094] mode=indexing
          tunnel: w6051 -> [w6095]
          tunnel: [w6091] -> w6054 mode=indexing
          n2730 = Unbundle By Name(w6094) -> ("command"=w6093:string, "command data"=w6092:variant)
          n2731 = call "App enquece.vi"("command data"=w6092, "command"=w6093, "queue in"=w6095) -> ("error out"=w6091:errorcluster)  [unwired: 7 in, 1 out]
        }
        n2732 = Merge Errors(w6055, w6054) -> (w6053:errorcluster)
      }
      frame "Test DRV 8A" {
        w6102 = T11 {"command"="", "command data"=variant} ("element")
        w6096 = 8 ("DUT index(0-59)")
        w6128 = T11 {"command"="", "command data"=variant} ("element")
        n2733 = disable-structure shown="LOGGING==TRUE" {
          disable-tunnel: w6106 -> [w6144 _]
          frame condition #0 (active) {
            n2734 = Empty String/Path?(string/path=w6144) -> (empty?=w6147:bool)
            n2735 = Select(t="Quece timeout", s=w6147, f=w6144) -> (s? t:f=w6143:string)
            n2736 = call "string log (SubVI).vi"("Enum"=enum16{"Init", "Log", "Read"}."Log", "state Name"=w6143) -> ()  [unwired: 8 in, 2 out]
          }
          frame condition #1 {
          }
        }
        n2737 = Flush Queue(queue=w6107) -> (queue out=w6108:refnum<queue>)  [unwired: 1 in, 2 out]
        n2738 = Decrement(x=w6096) -> (x-1=w6100:i32)
        n2739 = Index Array(array=w6097, index=w6100) -> (element=w6098:refnum<vi>)
        n2740 = property class="ColBox"(reference=w6098, "Value"=u32 10000536 ("DRV 1")) -> ()  [unwired: 1 in, 2 out]
        n2741 = To Variant(anything=bool[] [FALSE, TRUE, FALSE, FALSE, FALSE, FALSE]) -> (Variant=w6125:variant)
        n2742 = To Variant(anything=T6."demux1_10_channel2" ("demux1_10(x6)_encode")) -> (Variant=w6129:variant)
        n2743 = To Variant(anything=T4."mux6_1_channel2_3" ("mux6_1(3wires)_encode")) -> (Variant=w6133:variant)
        n2744 = To Variant(anything=T5."mux10_1_channel2" ("mux10_1(x6)_encode")) -> (Variant=w6135:variant)
        n2745 = Bundle By Name(cluster=w6128, "command"="MEAS.mux10-1", "command data"=w6135) -> (w6123:T11)
        n2746 = Bundle By Name(cluster=w6128, "command"="MEAS.mux6_1", "command data"=w6133) -> (w6122:T11)
        n2747 = Bundle By Name(cluster=w6128, "command"="MEAS.demux1-10", "command data"=w6129) -> (w6121:T11)
        n2748 = Bundle By Name(cluster=w6128, "command"="MEAS.eMIC", "command data"=w6125) -> (w6120:T11)
        n2749 = Bundle By Name(cluster=w6128, "command"="MEAS.AllRelaysOFF") -> (w6124:T11)
        n2750 = Build Array(w6124, w6123, w6122, w6121, w6120) -> (w6115:T11[])
        n2751 = Bundle By Name(cluster=w6102, "command"="MEAS.requestAC", "command data"=w6096) -> (w6116:T11)
        n2752 = Bundle By Name(cluster=w6102, "command"="Apps.WaitForEvent", "command data"=w6096) -> (w6101:T11)
        n2753 = Bundle By Name(cluster=w6102, "command"="MEAS.DMM dual read") -> (w6117:T11)
        n2754 = Bundle By Name(cluster=w6102, "command"="Apps.UI Update 1") -> (w6103:T11)
        n2755 = Build Array(w6117, w6116, w6101, w6103) -> (w6114:T11[])
        n2756 = Build Array (concatenate)(w6115, w6114) -> (w6113:T11[])
        n2757 = for {
          tunnel: w6113 -> [w6151] mode=indexing
          tunnel: w6108 -> [w6152]
          tunnel: [w6148] -> w6111 mode=indexing
          n2758 = Unbundle By Name(w6151) -> ("command"=w6150:string, "command data"=w6149:variant)
          n2759 = call "App enquece.vi"("command data"=w6149, "command"=w6150, "queue in"=w6152) -> ("error out"=w6148:errorcluster)  [unwired: 7 in, 1 out]
        }
        n2760 = Merge Errors(w6112, w6111) -> (w6110:errorcluster)
      }
      frame "Test DRV 9A" {
        w6159 = T11 {"command"="", "command data"=variant} ("element")
        w6153 = 9 ("DUT index(0-59)")
        w6185 = T11 {"command"="", "command data"=variant} ("element")
        n2761 = disable-structure shown="LOGGING==TRUE" {
          disable-tunnel: w6163 -> [w6201 _]
          frame condition #0 (active) {
            n2762 = Empty String/Path?(string/path=w6201) -> (empty?=w6204:bool)
            n2763 = Select(t="Quece timeout", s=w6204, f=w6201) -> (s? t:f=w6200:string)
            n2764 = call "string log (SubVI).vi"("Enum"=enum16{"Init", "Log", "Read"}."Log", "state Name"=w6200) -> ()  [unwired: 8 in, 2 out]
          }
          frame condition #1 {
          }
        }
        n2765 = Flush Queue(queue=w6164) -> (queue out=w6165:refnum<queue>)  [unwired: 1 in, 2 out]
        n2766 = Decrement(x=w6153) -> (x-1=w6157:i32)
        n2767 = Index Array(array=w6154, index=w6157) -> (element=w6155:refnum<vi>)
        n2768 = property class="ColBox"(reference=w6155, "Value"=u32 10000536 ("DRV 1")) -> ()  [unwired: 1 in, 2 out]
        n2769 = To Variant(anything=bool[] [FALSE, FALSE, TRUE, FALSE, FALSE, FALSE]) -> (Variant=w6182:variant)
        n2770 = To Variant(anything=T6."demux1_10_channel2" ("demux1_10(x6)_encode")) -> (Variant=w6186:variant)
        n2771 = To Variant(anything=T4."mux6_1_channel3_3" ("mux6_1(3wires)_encode")) -> (Variant=w6190:variant)
        n2772 = To Variant(anything=T5."mux10_1_channel2" ("mux10_1(x6)_encode")) -> (Variant=w6192:variant)
        n2773 = Bundle By Name(cluster=w6185, "command"="MEAS.mux10-1", "command data"=w6192) -> (w6180:T11)
        n2774 = Bundle By Name(cluster=w6185, "command"="MEAS.mux6_1", "command data"=w6190) -> (w6179:T11)
        n2775 = Bundle By Name(cluster=w6185, "command"="MEAS.demux1-10", "command data"=w6186) -> (w6178:T11)
        n2776 = Bundle By Name(cluster=w6185, "command"="MEAS.eMIC", "command data"=w6182) -> (w6177:T11)
        n2777 = Bundle By Name(cluster=w6185, "command"="MEAS.AllRelaysOFF") -> (w6181:T11)
        n2778 = Build Array(w6181, w6180, w6179, w6178, w6177) -> (w6172:T11[])
        n2779 = Bundle By Name(cluster=w6159, "command"="MEAS.requestAC", "command data"=w6153) -> (w6173:T11)
        n2780 = Bundle By Name(cluster=w6159, "command"="Apps.WaitForEvent", "command data"=w6153) -> (w6158:T11)
        n2781 = Bundle By Name(cluster=w6159, "command"="MEAS.DMM dual read") -> (w6174:T11)
        n2782 = Bundle By Name(cluster=w6159, "command"="Apps.UI Update 1") -> (w6160:T11)
        n2783 = Build Array(w6174, w6173, w6158, w6160) -> (w6171:T11[])
        n2784 = Build Array (concatenate)(w6172, w6171) -> (w6170:T11[])
        n2785 = for {
          tunnel: w6170 -> [w6208] mode=indexing
          tunnel: w6165 -> [w6209]
          tunnel: [w6205] -> w6168 mode=indexing
          n2786 = Unbundle By Name(w6208) -> ("command"=w6207:string, "command data"=w6206:variant)
          n2787 = call "App enquece.vi"("command data"=w6206, "command"=w6207, "queue in"=w6209) -> ("error out"=w6205:errorcluster)  [unwired: 7 in, 1 out]
        }
        n2788 = Merge Errors(w6169, w6168) -> (w6167:errorcluster)
      }
      frame "Test DRV 10A" {
        w6216 = T11 {"command"="", "command data"=variant} ("element")
        w6210 = 10 ("DUT index(0-59)")
        w6242 = T11 {"command"="", "command data"=variant} ("element")
        n2789 = disable-structure shown="LOGGING==TRUE" {
          disable-tunnel: w6220 -> [w6258 _]
          frame condition #0 (active) {
            n2790 = Empty String/Path?(string/path=w6258) -> (empty?=w6261:bool)
            n2791 = Select(t="Quece timeout", s=w6261, f=w6258) -> (s? t:f=w6257:string)
            n2792 = call "string log (SubVI).vi"("Enum"=enum16{"Init", "Log", "Read"}."Log", "state Name"=w6257) -> ()  [unwired: 8 in, 2 out]
          }
          frame condition #1 {
          }
        }
        n2793 = Flush Queue(queue=w6221) -> (queue out=w6222:refnum<queue>)  [unwired: 1 in, 2 out]
        n2794 = Decrement(x=w6210) -> (x-1=w6214:i32)
        n2795 = Index Array(array=w6211, index=w6214) -> (element=w6212:refnum<vi>)
        n2796 = property class="ColBox"(reference=w6212, "Value"=u32 10000536 ("DRV 1")) -> ()  [unwired: 1 in, 2 out]
        n2797 = To Variant(anything=bool[] [FALSE, FALSE, FALSE, TRUE, FALSE, FALSE]) -> (Variant=w6239:variant)
        n2798 = To Variant(anything=T6."demux1_10_channel2" ("demux1_10(x6)_encode")) -> (Variant=w6243:variant)
        n2799 = To Variant(anything=T4."mux6_1_channel4_3" ("mux6_1(3wires)_encode")) -> (Variant=w6247:variant)
        n2800 = To Variant(anything=T5."mux10_1_channel2" ("mux10_1(x6)_encode")) -> (Variant=w6249:variant)
        n2801 = Bundle By Name(cluster=w6242, "command"="MEAS.mux10-1", "command data"=w6249) -> (w6237:T11)
        n2802 = Bundle By Name(cluster=w6242, "command"="MEAS.mux6_1", "command data"=w6247) -> (w6236:T11)
        n2803 = Bundle By Name(cluster=w6242, "command"="MEAS.demux1-10", "command data"=w6243) -> (w6235:T11)
        n2804 = Bundle By Name(cluster=w6242, "command"="MEAS.eMIC", "command data"=w6239) -> (w6234:T11)
        n2805 = Bundle By Name(cluster=w6242, "command"="MEAS.AllRelaysOFF") -> (w6238:T11)
        n2806 = Build Array(w6238, w6237, w6236, w6235, w6234) -> (w6229:T11[])
        n2807 = Bundle By Name(cluster=w6216, "command"="MEAS.requestAC", "command data"=w6210) -> (w6230:T11)
        n2808 = Bundle By Name(cluster=w6216, "command"="Apps.WaitForEvent", "command data"=w6210) -> (w6215:T11)
        n2809 = Bundle By Name(cluster=w6216, "command"="MEAS.DMM dual read") -> (w6231:T11)
        n2810 = Bundle By Name(cluster=w6216, "command"="Apps.UI Update 1") -> (w6217:T11)
        n2811 = Build Array(w6231, w6230, w6215, w6217) -> (w6228:T11[])
        n2812 = Build Array (concatenate)(w6229, w6228) -> (w6227:T11[])
        n2813 = for {
          tunnel: w6227 -> [w6265] mode=indexing
          tunnel: w6222 -> [w6266]
          tunnel: [w6262] -> w6225 mode=indexing
          n2814 = Unbundle By Name(w6265) -> ("command"=w6264:string, "command data"=w6263:variant)
          n2815 = call "App enquece.vi"("command data"=w6263, "command"=w6264, "queue in"=w6266) -> ("error out"=w6262:errorcluster)  [unwired: 7 in, 1 out]
        }
        n2816 = Merge Errors(w6226, w6225) -> (w6224:errorcluster)
      }
      frame "Test DRV 11A" {
        w6273 = T11 {"command"="", "command data"=variant} ("element")
        w6267 = 11 ("DUT index(0-59)")
        w6299 = T11 {"command"="", "command data"=variant} ("element")
        n2817 = disable-structure shown="LOGGING==TRUE" {
          disable-tunnel: w6277 -> [w6315 _]
          frame condition #0 (active) {
            n2818 = Empty String/Path?(string/path=w6315) -> (empty?=w6318:bool)
            n2819 = Select(t="Quece timeout", s=w6318, f=w6315) -> (s? t:f=w6314:string)
            n2820 = call "string log (SubVI).vi"("Enum"=enum16{"Init", "Log", "Read"}."Log", "state Name"=w6314) -> ()  [unwired: 8 in, 2 out]
          }
          frame condition #1 {
          }
        }
        n2821 = Flush Queue(queue=w6278) -> (queue out=w6279:refnum<queue>)  [unwired: 1 in, 2 out]
        n2822 = Decrement(x=w6267) -> (x-1=w6271:i32)
        n2823 = Index Array(array=w6268, index=w6271) -> (element=w6269:refnum<vi>)
        n2824 = property class="ColBox"(reference=w6269, "Value"=u32 10000536 ("DRV 1")) -> ()  [unwired: 1 in, 2 out]
        n2825 = To Variant(anything=bool[] [FALSE, FALSE, FALSE, FALSE, TRUE, FALSE]) -> (Variant=w6296:variant)
        n2826 = To Variant(anything=T6."demux1_10_channel2" ("demux1_10(x6)_encode")) -> (Variant=w6300:variant)
        n2827 = To Variant(anything=T4."mux6_1_channel5_3" ("mux6_1(3wires)_encode")) -> (Variant=w6304:variant)
        n2828 = To Variant(anything=T5."mux10_1_channel2" ("mux10_1(x6)_encode")) -> (Variant=w6306:variant)
        n2829 = Bundle By Name(cluster=w6299, "command"="MEAS.mux10-1", "command data"=w6306) -> (w6294:T11)
        n2830 = Bundle By Name(cluster=w6299, "command"="MEAS.mux6_1", "command data"=w6304) -> (w6293:T11)
        n2831 = Bundle By Name(cluster=w6299, "command"="MEAS.demux1-10", "command data"=w6300) -> (w6292:T11)
        n2832 = Bundle By Name(cluster=w6299, "command"="MEAS.eMIC", "command data"=w6296) -> (w6291:T11)
        n2833 = Bundle By Name(cluster=w6299, "command"="MEAS.AllRelaysOFF") -> (w6295:T11)
        n2834 = Build Array(w6295, w6294, w6293, w6292, w6291) -> (w6286:T11[])
        n2835 = Bundle By Name(cluster=w6273, "command"="MEAS.requestAC", "command data"=w6267) -> (w6287:T11)
        n2836 = Bundle By Name(cluster=w6273, "command"="Apps.WaitForEvent", "command data"=w6267) -> (w6272:T11)
        n2837 = Bundle By Name(cluster=w6273, "command"="MEAS.DMM dual read") -> (w6288:T11)
        n2838 = Bundle By Name(cluster=w6273, "command"="Apps.UI Update 1") -> (w6274:T11)
        n2839 = Build Array(w6288, w6287, w6272, w6274) -> (w6285:T11[])
        n2840 = Build Array (concatenate)(w6286, w6285) -> (w6284:T11[])
        n2841 = for {
          tunnel: w6284 -> [w6322] mode=indexing
          tunnel: w6279 -> [w6323]
          tunnel: [w6319] -> w6282 mode=indexing
          n2842 = Unbundle By Name(w6322) -> ("command"=w6321:string, "command data"=w6320:variant)
          n2843 = call "App enquece.vi"("command data"=w6320, "command"=w6321, "queue in"=w6323) -> ("error out"=w6319:errorcluster)  [unwired: 7 in, 1 out]
        }
        n2844 = Merge Errors(w6283, w6282) -> (w6281:errorcluster)
      }
      frame "Test DRV 12A" {
        w6330 = T11 {"command"="", "command data"=variant} ("element")
        w6324 = 12 ("DUT index(0-59)")
        w6356 = T11 {"command"="", "command data"=variant} ("element")
        n2845 = disable-structure shown="LOGGING==TRUE" {
          disable-tunnel: w6334 -> [w6372 _]
          frame condition #0 (active) {
            n2846 = Empty String/Path?(string/path=w6372) -> (empty?=w6375:bool)
            n2847 = Select(t="Quece timeout", s=w6375, f=w6372) -> (s? t:f=w6371:string)
            n2848 = call "string log (SubVI).vi"("Enum"=enum16{"Init", "Log", "Read"}."Log", "state Name"=w6371) -> ()  [unwired: 8 in, 2 out]
          }
          frame condition #1 {
          }
        }
        n2849 = Flush Queue(queue=w6335) -> (queue out=w6336:refnum<queue>)  [unwired: 1 in, 2 out]
        n2850 = Decrement(x=w6324) -> (x-1=w6328:i32)
        n2851 = Index Array(array=w6325, index=w6328) -> (element=w6326:refnum<vi>)
        n2852 = property class="ColBox"(reference=w6326, "Value"=u32 10000536 ("DRV 1")) -> ()  [unwired: 1 in, 2 out]
